vi "Average tau0.vi"(8 "error in":errorcluster, 9 "# of shots":i32, 10 "extParam":T1={"Tau"=nan, "Tau0cor"=nan, "ext"=nan, "extCorr"=nan, "stdevTau"=nan, "eTau"=nan, "taucorr"=nan, "Tau0"=nan, "max"=nan}, 11 "CRDS Cell in":refnum<class "CRDS Cell.lvclass">) -> (0 "error out":errorcluster, 3 "CRDS Cell out":refnum<class "CRDS Cell.lvclass">)   [LabVIEW 2016, in "CRDS Lib.lvlib" / "CRDS Cell.lvclass"]
doc: "Average taus recorded on filter to give a mean tau0. The values tau0 and tau0cor will be averaged over the number of times this vi is called or the value of <b># of shots</b>, whichever is smaller.\n\nOnly accessors can throw errors here."
uses:
  CRDS Cell.lvclass
  extParam Ctl.ctl
  CRDS Cell.lvclass/CRDS Cell.ctl
  Data/Cell/CRDS Cell Data.lvclass/CRDS Cell Data.ctl
  <vilib>/Analysis/baseanly.llb/Mean (DBL).vi
  Read Data.vi
  Data/Cell/Write extParam.vi
  Write Data.vi
  Write tau_0.vi
  Write corr tau0.vi
  Data/Cell/CRDS Cell Data.lvclass
  <vilib>/Analysis/NI_AALBase.lvlib
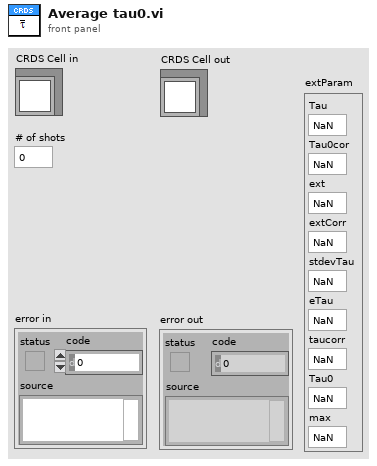
[diagram p1: front panel]
types:
  T1 = typedef "CRDS Lib.lvlib/CRDS Cell Data.lvclass/extParam Ctl.ctl" = cluster{"Tau":sgl, "Tau0cor":sgl, "ext":sgl, "extCorr":sgl, "stdevTau":sgl, "eTau":sgl, "taucorr":sgl, "Tau0":sgl, "max":sgl}
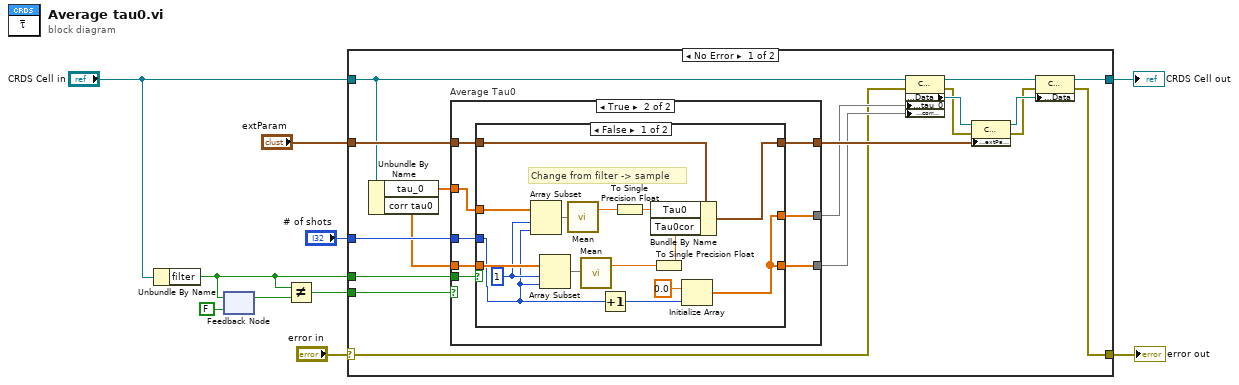
[diagram p0: block diagram]
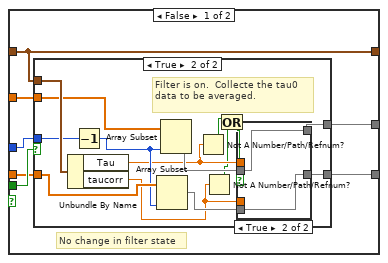
[diagram p2: hidden frame]
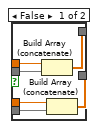
[diagram p4: hidden frame]
diagram:
  n1 = Unbundle By Name("CRDS Cell in") -> ("filter"=w3:bool)
  n2 = feedback-in #1(w3) -> ()
  n3 = feedback #1(FALSE ("filter")) -> (w4:bool)
  n4 = Not Equal?(x=w3, y=w4) -> (x != y?=w1:bool)
  n5 = case shown="No Error" "error in" {
    selector: "error in" -> [w15 w87]
    tunnel: [w12 w87] -> w9
    tunnel: [w21 w86] -> w8
    tunnel: "CRDS Cell in" -> [w20 w86]
    tunnel: "extParam" -> [w28 _]
    tunnel: "# of shots" -> [w27 _]
    tunnel: w3 -> [w26 _]
    tunnel: w1 -> [w11 _]
    frame No Error {
      n6 = Unbundle By Name(w20) -> ("tau_0"=w19:dbl[], "corr tau0"=w18:dbl[])
      n7 = case "Average Tau0" shown="True" w11 {
        tunnel: w26 -> [w32 w67]
        tunnel: w28 -> [w35 w66]
        tunnel: [w35 w65] -> w24
        tunnel: w19 -> [w34 w64]
        tunnel: [w33 w63] -> w16
        tunnel: w18 -> [w31 w62]
        tunnel: [w30 w61] -> w17
        tunnel: w27 -> [w29 w60]
        frame False {
          # "No change in filter state"
          n8 = case shown="True" w32 {
            tunnel: w35 -> [_ w51]
            tunnel: w34 -> [w37 w48]
            tunnel: [w37 w50] -> w33
            tunnel: w31 -> [w36 w46]
            tunnel: [w36 w43] -> w30
            tunnel: w29 -> [_ w49]
            frame False {
              # "On sample."
            }
            frame True {
              # "Filter is on.  Collecte the tau0  data to be averaged."
              n9 = Unbundle By Name(w51) -> ("Tau"=w42:sgl, "taucorr"=w41:sgl)
              n10 = Decrement(x=w49) -> (x-1=w45:i32)
              n11 = Array Subset(array=w46, length=w45) -> (w44:dbl[])  [unwired: 1 in]
              n12 = Array Subset(array=w48, length=w45) -> (w47:dbl[])  [unwired: 1 in]
              n13 = Not A Number/Path/Refnum?(number/path/refnum=w42) -> (NaN/Path/Refnum?=w40:bool)
              n14 = Not A Number/Path/Refnum?(number/path/refnum=w41) -> (NaN/Path/Refnum?=w39:bool)
              n15 = Or(x=w40, y=w39) -> (x .or. y?=w38:bool)
              n16 = case shown="True" w38 {
                tunnel: w42 -> [w57 _]
                tunnel: [w56 w59] -> w50
                tunnel: w47 -> [w55 w59]
                tunnel: w44 -> [w54 w58]
                tunnel: w41 -> [w53 _]
                tunnel: [w52 w58] -> w43
                frame False {
                  n17 = Build Array (concatenate)(w57, w55) -> (w56:dbl[])
                  n18 = Build Array (concatenate)(w53, w54) -> (w52:dbl[])
                }
                frame True {
                }
              }
            }
          }
        }
        frame True {
          n19 = case shown="False" w67 {
            tunnel: w66 -> [w82 w85]
            tunnel: [w81 w85] -> w65
            tunnel: w64 -> [w73 w84]
            tunnel: [w75 w84] -> w63
            tunnel: w62 -> [w72 w83]
            tunnel: [w75 w83] -> w61
            tunnel: w60 -> [w70 _]
            frame False {
              w71 = 1 ("index")
              # "Change from filter -> sample"
              n20 = Array Subset(array=w73, index=w71, length=w70) -> (w69:dbl[])
              n21 = Array Subset(array=w72, index=w71, length=w70) -> (w68:dbl[])
              n22 = call-poly <vilib>:"Mean.vi"("X"=w69) -> ("mean"=w80:dbl)  [unwired: 1 out]
              n23 = call-poly <vilib>:"Mean.vi"("X"=w68) -> ("mean"=w78:dbl)  [unwired: 1 out]
              n24 = Increment(x=w70) -> (x+1=w74:i32)
              n25 = To Single Precision Float(number=w80) -> (single precision float=w79:sgl)
              n26 = To Single Precision Float(number=w78) -> (single precision float=w77:sgl)
              n27 = Bundle By Name(cluster=w82, "Tau0"=w79, "Tau0cor"=w77) -> (w81:T1)
              n28 = Initialize Array(0.0, w74) -> (w75:dbl[])
            }
            frame True {
              # "Change from sample -> filter. Do nothing, the matrices have already been zeroed."
            }
          }
        }
      }
      n29 = property class="CRDS Cell"(reference=w20, error in=w15, "Accessors:tau_0"=w16, "Accessors:corr tau0"=w17) -> (reference out=w23:refnum<class "CRDS Cell.lvclass">, error out=w14:errorcluster, "Accessors:Data"=w25:refnum<class "CRDS Cell Data.lvclass">)
      n30 = property class="CRDS Cell"(reference=w25, error in=w14, "Data Access:extParam"=w24) -> (reference out=w22:refnum<class "CRDS Cell Data.lvclass">, error out=w13:errorcluster)
      n31 = property class="CRDS Cell"(reference=w23, error in=w13, "Accessors:Data"=w22) -> (reference out=w21:refnum<class "CRDS Cell.lvclass">, error out=w12:errorcluster)
    }
    frame Error {
    }
  }
  "error out" <- w9
  "CRDS Cell out" <- w8
